vi "Get File Properties.vi"(7 "scope":T2, 8 "error in (no error)":errorcluster, 10 "owner":string, 11 "error list <top>":variant) -> (0 "error out":errorcluster, 2 "properties":T1, 3 "error list <top> dup":variant)   [LabVIEW 2017]
uses:
  Scope.ctl
  Error Code File Properties.ctl
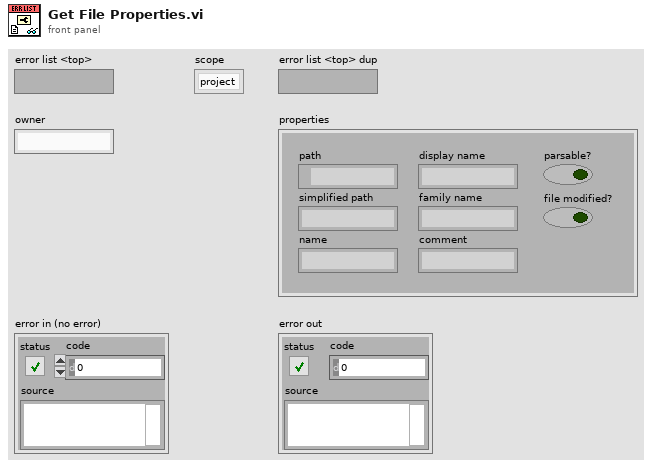
[diagram p1: front panel]
types:
  T1 = typedef "Error Code File Properties.ctl" = cluster{"path":path, "simplified path":string, "name":string, "display name":string, "family name":string, "comment":string, "parsable?":bool, "file modified?":bool}
  T2 = typedef "Scope.ctl" = enum16{"project", "global"}
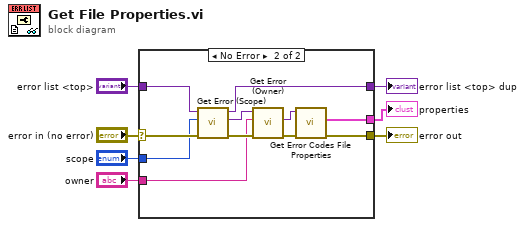
[diagram p0: block diagram]
diagram:
  n1 = case shown="No Error" "error in (no error)" {
    selector: "error in (no error)" -> [w9 w20]
    tunnel: "scope" -> [_ w15]
    tunnel: "error list <top>" -> [w8 w14]
    tunnel: [w8 w13] -> w5
    tunnel: "owner" -> [_ w12]
    tunnel: [_ w11] -> w3
    tunnel: [w9 w10] -> w1
    frame Error {
    }
    frame No Error {
      n2 = call "Get Error (Scope).vi"("error in (no error)"=w20, "scope"=w15, "error list <top>"=w14) -> ("error out"=w19:errorcluster, "error list <scope>"=w18:variant, "error list <top> dup"=w13:variant)  [unwired: 5 in, 1 out]
      n3 = call "Get Error (Owner).vi"("error in (no error)"=w19, "owner"=w12, "error list <scope>"=w18) -> ("error out"=w16:errorcluster, "error list <owner>"=w17:variant)  [unwired: 5 in, 2 out]
      n4 = call "Get Error Codes File Properties.vi"("error in (no error)"=w16, "error list <owner> in"=w17) -> ("error out"=w10:errorcluster, "properties"=w11:T1)  [unwired: 6 in, 2 out]
    }
  }
  "error list <top> dup" <- w5
  "properties" <- w3
  "error out" <- w1
